vi "Basic Set Entry Mode.vi"(6 "chip select  (1st chip)":enum16{"1st chip", "2nd chip"}(ring), 8 "error in (no error)":errorcluster, 10 "entry mode (increment & no shift)":T2(ring), 11 "cluster of private data in":T1={"FPGA VI Reference"=refnum, "device index"=0, "screen size"=enum."8x1", "font size"=enum."5x8", "auto wrap"=FALSE, "alignment"=enum."None", "number of line"=enum."2 lines", "shift 0"=0, "entry mode 0"=enum."increment & no shift", "shift 1"=0, "entry mode 1"=enum."increment & no shift"}) -> (0 "error out":errorcluster, 3 "cluster of private data out":T1={"FPGA VI Reference"=refnum, "device index"=0, "screen size"=enum."8x1", "font size"=enum."5x8", "auto wrap"=FALSE, "alignment"=enum."None", "number of line"=enum."2 lines", "shift 0"=0, "entry mode 0"=enum."increment & no shift", "shift 1"=0, "entry mode 1"=enum."increment & no shift"})   [LabVIEW 2017, in "HD44780.lvclass"]
uses:
  HD44780.lvclass
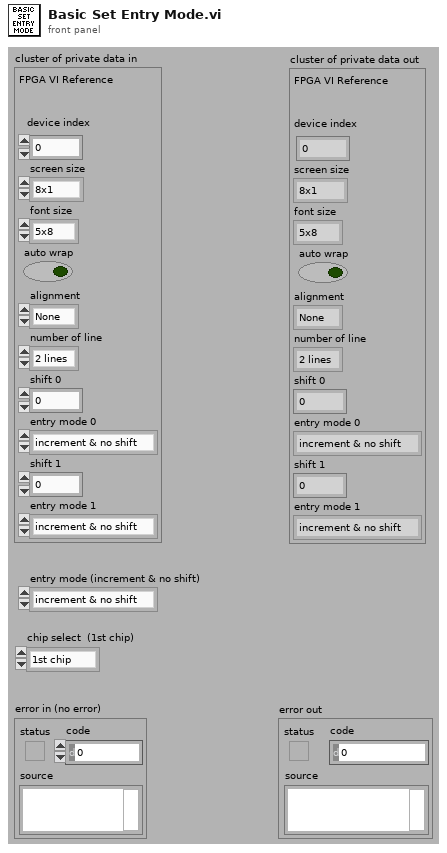
[diagram p1: front panel]
types:
  T1 = cluster{"FPGA VI Reference":refnum<k20>, "device index":i8, "screen size":enum8{"8x1", "8x2", "12x4", "16x1", "16x2", "16x4", "20x1", "20x2", "20x4", "24x1", "24x2", "40x2", "40x4"}, "font size":enum8{"5x8", "5x10"}, "auto wrap":bool, "alignment":enum16{"None", "Left", "Center", "Right"}, "number of line":enum8{"1 line", "2 lines"}, "shift 0":i8, "entry mode 0":enum8{"increment & no shift", "increment & shift", "decrement & no shift", "decrement & shift"}, "shift 1":i8, "entry mode 1":enum8{"increment & no shift", "increment & shift", "decrement & no shift", "decrement & shift"}}
  T2 = enum8{"increment & no shift", "increment & shift", "decrement & no shift", "decrement & shift"}
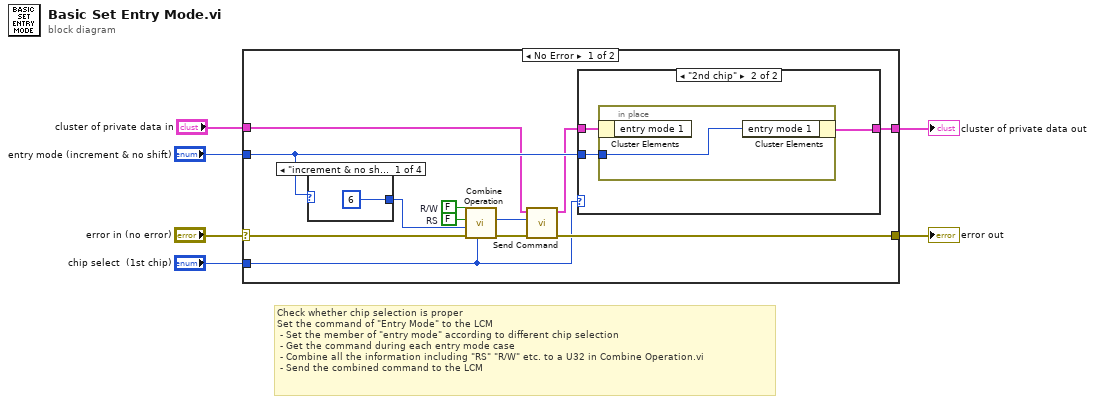
[diagram p0: block diagram]
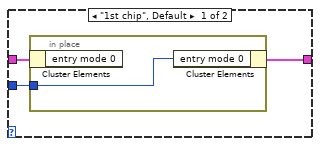
[diagram p2: hidden frame]
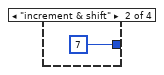
[diagram p3: hidden frame]
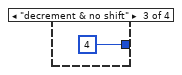
[diagram p4: hidden frame]
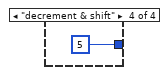
[diagram p5: hidden frame]
diagram:
  # "Check whether chip selection is proper\nSet the command of \"Entry Mode\" to the LCM\n - Set the member of \"entry mode\" according to different chip selection\n - Get the command during each entry mode case\n - Combine all the information including \"RS\" \"R/W\" etc. to a U32 in Combine Operation.vi \n - Send the combined command to the LCM"
  n1 = case shown="No Error" "error in (no error)" {
    selector: "error in (no error)" -> [w8 w32]
    tunnel: [w15 w31] -> w6
    tunnel: [w14 w32] -> w5
    tunnel: "entry mode (increment & no shift)" -> [w11 _]
    tunnel: "cluster of private data in" -> [w10 w31]
    tunnel: "chip select  (1st chip)" -> [w7 _]
    frame No Error {
      w12 = FALSE  # RS
      w13 = FALSE  # R/W
      n2 = case shown="\"increment & no shift\", Default" w11 {
        tunnel: [u8 6 u8 7 u8 4 u8 5] -> w18
        frame "increment & no shift", Default {
        }
        frame "increment & shift" {
        }
        frame "decrement & no shift" {
        }
        frame "decrement & shift" {
        }
      }
      n3 = call "Combine Operation.vi"("chip select  (1st chip)"=w7, "error in (no error)"=w8, "cmd/data"=w18, "RS"=w12, "R/W"=w13) -> ("error out"=w17:errorcluster, "output"=w16:u32)  [unwired: 5 in]
      n4 = call "Send Command.vi"("error in (no error)"=w17, "operation"=w16, "cluster of private data in"=w10) -> ("error out"=w14:errorcluster, "cluster of private data out"=w9:T1)  [unwired: 6 in, 1 out]
      n5 = case shown="\"2nd chip\"" w7 {
        tunnel: w9 -> [w21 w25]
        tunnel: w11 -> [w20 w24]
        tunnel: [w19 w23] -> w15
        frame "1st chip", Default {
          n6 = in-place {
            in-place-border: w20 -> [w22]
            n7 = in-place-cluster #1(w21) -> ()  [unwired: 1 out]
            n8 = in-place-cluster #1("entry mode 0"=w22) -> (w19:T1)
          }
        }
        frame "2nd chip" {
          n9 = in-place {
            in-place-border: w24 -> [w26]
            n10 = in-place-cluster #2(w25) -> ()  [unwired: 1 out]
            n11 = in-place-cluster #2("entry mode 1"=w26) -> (w23:T1)
          }
        }
      }
    }
    frame Error {
    }
  }
  "cluster of private data out" <- w6
  "error out" <- w5
